vi "Focus Initialize.vi"(8 "error in (no error)":errorcluster, 10 "Motion Settings":T1, 11 "Focus Class in":refnum<class "Focus Class.lvclass">) -> (0 "error out":errorcluster, 1 "Motor Positions":i32[](array[numeric]), 2 "Device Name":string, 3 "Focus Class out":refnum<class "Focus Class.lvclass">)   [LabVIEW 2021, in "Focus Class.lvclass"]
uses:
  Focus Class.lvclass
  Focus cluster Motion Settings.ctl
  Focus Class.lvclass/Focus Class.ctl
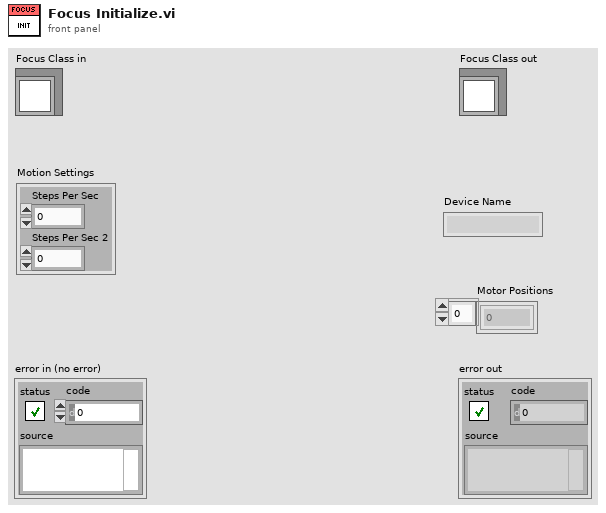
[diagram p1: front panel]
types:
  T1 = typedef "Focus cluster Motion Settings.ctl" = cluster{"Steps Per Sec":i32, "Steps Per Sec 2":i32}
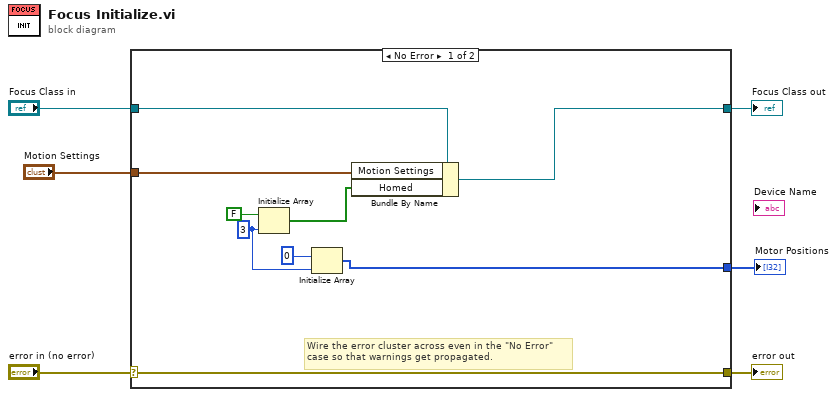
[diagram p0: block diagram]
diagram:
  n1 = case shown="No Error" "error in (no error)" {
    selector: "error in (no error)" -> [w15 w17]
    tunnel: [w15 w17] -> w5
    tunnel: [w13 w16] -> w3
    tunnel: "Focus Class in" -> [w12 w16]
    tunnel: "Motion Settings" -> [w14 _]
    tunnel: [w7 _] -> w1
    frame No Error {
      w9 = 3 ("dimension size")
      # "Wire the error cluster across even in the \"No Error\"\ncase so that warnings get propagated."
      n2 = Initialize Array(FALSE, w9) -> (w10:bool[])
      n3 = Initialize Array(0 ("dimension size"), w9) -> (w7:i32[])
      n4 = Bundle By Name(cluster=w12, "Motion Settings"=w14, "Homed"=w10) -> (w13:refnum<class "Focus Class.lvclass">)
    }
    frame Error {
    }
  }
  "error out" <- w5
  "Focus Class out" <- w3
  "Motor Positions" <- w1
